vi "LOOP_pp3c_loadNext.vi"(0 "State Info In":T8={"Curr  tr"=0, "Curr (ms)"=0, "Cum (ms)"=0, "Run loop diff"=0, "Tone countdown (ms)"=0, "Countdown (ms)"=0, "Curr State"=enum."0 NULL", "Prev State"=enum."1 Habituation", "Rw"=FALSE, "Sw"=FALSE, "Tone\nGate"=FALSE, "Punish"=FALSE, "Current DAQ DO Int"=0, "Current Loaded Trial"={"Trial Type Number"=1, "Trial Type"=enum."GO", "Trial Weight"=100, "Shock (mA)"=0.3, "Duration (ms)"=0.25, "Sound Type"=enum."04 FM Sweep", "Stim P1"=4000.0, "Stim P2"=0.0, "Stim P3"=0.0, "Stim P4"=2000.0, "DAQ Amplitude (V)"=0.25}, "Total trials memo"=0, "State start cum memo (ms)"=0, "Last dur jump time memo (ms)"=0, "Last dur shock time memo (ms)"=0, "Tone repeat memo (ms)"=0, "Webcam on"=FALSE, "Webcam recording"=FALSE, "State update flag"=FALSE, "Last loaded shock voltage"=0.0, "Vid upd"=enum."0", "First time tone"=FALSE} {"Current DAQ DO Int" format="%016b"; "Current Loaded Trial"."DAQ Amplitude (V)" min=0.0 max=5.0 format="%_4g"; "Current Loaded Trial"."Shock (mA)" min=-1.0 max=5.0; "Current Loaded Trial"."Trial Weight" step=1; "Current Loaded Trial"."Duration (ms)" min=0.0 max=1.0; "Current Loaded Trial"."Trial Type Number" min=1 max=256 step=1}, 1 "Session param (dynamic)":T7={"Def M shock (uA)"=400.0, "Def F shock (uA)"=0.0}, 2 "Session List (Hidden variable)":u8[](array[numeric]), 3 "Trial Types":T1[](array[typedef])=[{"Trial Type Number"=1, "Trial Type"=enum."GO", "Trial Weight"=1, "Shock (mA)"=-1.0, "Duration (ms)"=250.0, "Sound Type"=enum."04 FM Sweep", "Stim P1"=4000.0, "Stim P2"=0.0, "Stim P3"=0.0, "Stim P4"=2000.0, "DAQ Amplitude (V)"=0.25}, {"Trial Type Number"=2, "Trial Type"=enum."NOGO", "Trial Weight"=1, "Shock (mA)"=-1.0, "Duration (ms)"=250.0, "Sound Type"=enum."04 FM Sweep", "Stim P1"=2000.0, "Stim P2"=0.0, "Stim P3"=0.0, "Stim P4"=4000.0, "DAQ Amplitude (V)"=0.25}] {"DAQ Amplitude (V)" min=0.0 max=5.0 format="%_4g"; "Shock (mA)" min=-1.0 max=5.0; "Trial Weight" step=1; "Duration (ms)" min=0.0 max=1.0; "Trial Type Number" min=1 max=256 step=1}, 5 "Daq config In":T4={"Sound AO"="Dev6/ao0", "Shock intesity AO"="Dev6/ao1", "Code_LED DO"="Dev6/port1:2", "Switch DI"="Dev6/port1/line0", "Webcam"="cam9", "Sound AO task"="", "Sound card task"=0, "Shock intensity AO task"="", "Code_LED DO task"="", "Switch DI task"="", "AO <=> Sound card"=FALSE, "Sound card"=0, "sample rate"=100000.0, "Variable shock"=TRUE, "Webcam on"=FALSE, "Waveform memo"={"t0"=timestamp(0 s since 1904-01-01), "dt"=1.0, "Y"=[]}, "Tone trigger"="PFI1", "Master-9 DO"="", "Master-9 DO task"="Dev6/port0/line5:7"} {"sample rate" min=8000.0; "Sound card task" format="%.0x"}, 7 "log queue in":refnum<queue>, 11 "error in (no error)":errorcluster) -> (4 "State Info Out":T8={"Curr  tr"=0, "Curr (ms)"=0, "Cum (ms)"=0, "Run loop diff"=0, "Tone countdown (ms)"=0, "Countdown (ms)"=0, "Curr State"=enum."0 NULL", "Prev State"=enum."1 Habituation", "Rw"=FALSE, "Sw"=FALSE, "Tone\nGate"=FALSE, "Punish"=FALSE, "Current DAQ DO Int"=0, "Current Loaded Trial"={"Trial Type Number"=1, "Trial Type"=enum."GO", "Trial Weight"=100, "Shock (mA)"=0.3, "Duration (ms)"=0.25, "Sound Type"=enum."04 FM Sweep", "Stim P1"=4000.0, "Stim P2"=0.0, "Stim P3"=0.0, "Stim P4"=2000.0, "DAQ Amplitude (V)"=0.25}, "Total trials memo"=0, "State start cum memo (ms)"=0, "Last dur jump time memo (ms)"=0, "Last dur shock time memo (ms)"=0, "Tone repeat memo (ms)"=0, "Webcam on"=FALSE, "Webcam recording"=FALSE, "State update flag"=FALSE, "Last loaded shock voltage"=0.0, "Vid upd"=enum."0", "First time tone"=FALSE} {"Current DAQ DO Int" format="%016b"; "Current Loaded Trial"."DAQ Amplitude (V)" min=0.0 max=5.0 format="%_4g"; "Current Loaded Trial"."Shock (mA)" min=-1.0 max=5.0; "Current Loaded Trial"."Trial Weight" step=1; "Current Loaded Trial"."Duration (ms)" min=0.0 max=1.0; "Current Loaded Trial"."Trial Type Number" min=1 max=256 step=1}, 8 "log queue out":refnum<queue>, 15 "error out":errorcluster)   [LabVIEW 2013]
doc: "This VI loads the next trial into \"current loaded trial\" in the State info, and applies approrpiate variable shock if applicable"
uses:
  CTL_pp3c_LoopState.ctl
  pp3_CTL_BehavioralState.ctl
  pp3_CTL_Trial.ctl
  pp3_CTL_TrialType.ctl
  labolabo2/waveforms/WFTypes.ctl
  pp3_CTL_SessionParamDynamic.ctl
  CTL_pp3c_DaqStatus.ctl
  <vilib>/userdefined/High Color/IMAQdx.ctl
  <vilib>/sound2/lvsound2.llb/Sound Output Task ID.ctl
  <vilib>/DAQmx/write.llb/DAQmx Write (Analog 1D DBL 1Chan NSamp).vi
  <vilib>/DAQmx/create/channels.llb/DAQmx Create Channel (AO-Voltage-Basic).vi
  <vilib>/DAQmx/configure/timing.llb/DAQmx Timing (Sample Clock).vi
  <vilib>/DAQmx/miscellaneous.llb/DAQmx Fill In Error Info.vi
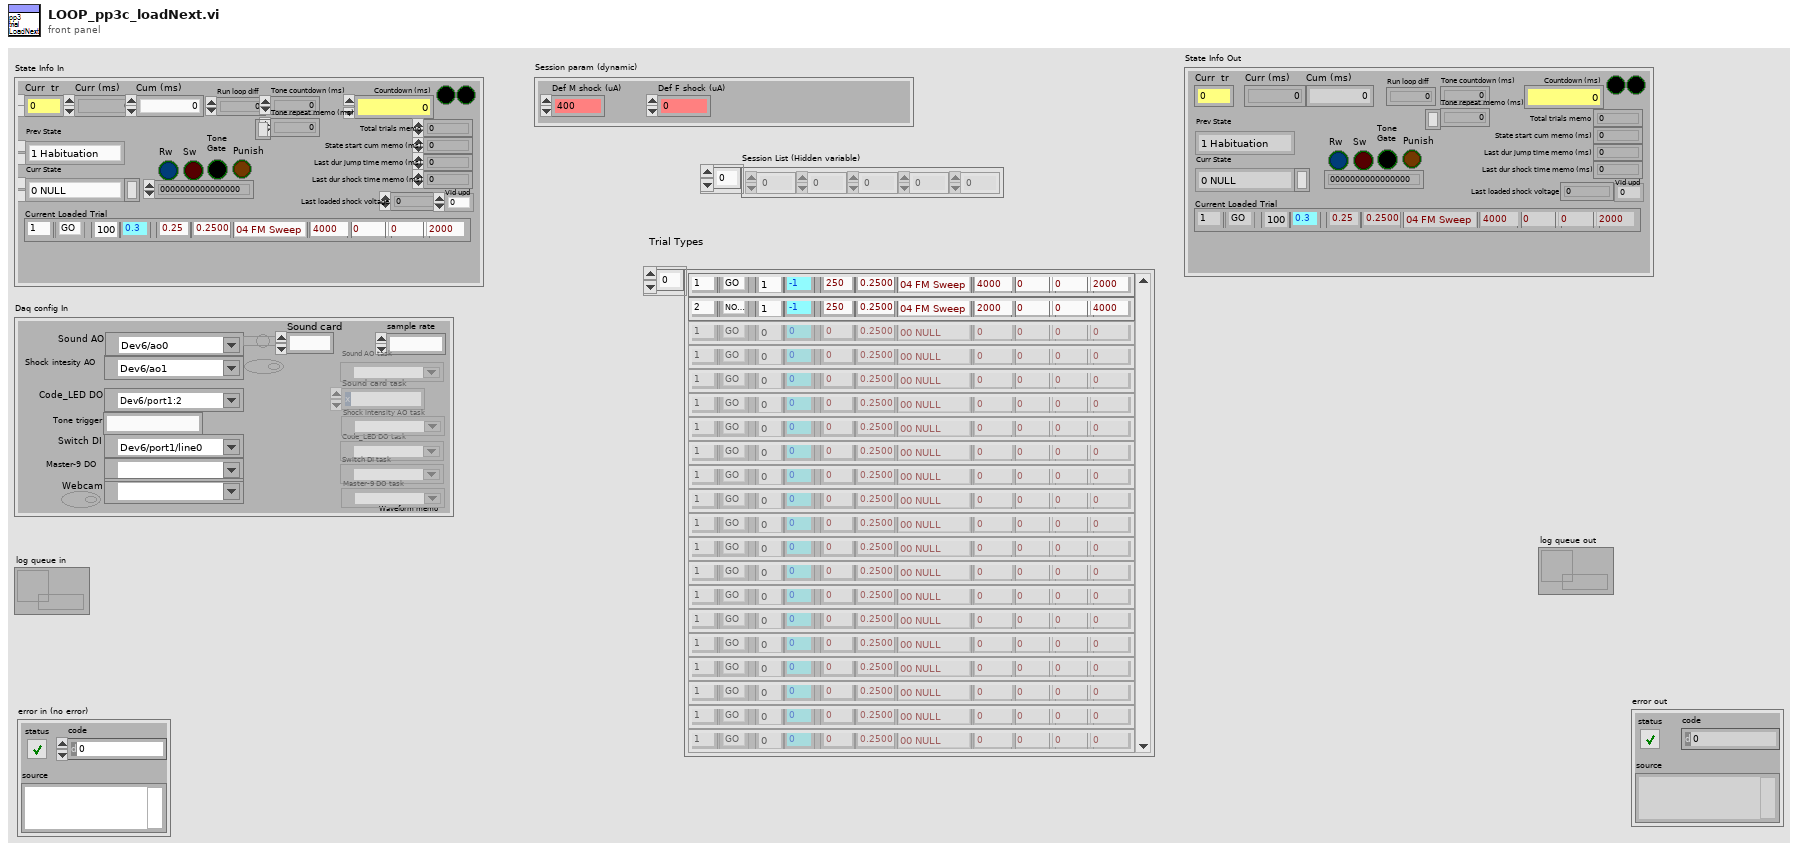
[diagram p1: front panel]
types:
  T1 = typedef "pp3_CTL_Trial.ctl" = cluster{"Trial Type Number":i16, "Trial Type":T2, "Trial Weight":u32, "Shock (mA)":dbl, "Duration (ms)":dbl, "Sound Type":T3, "Stim P1":dbl, "Stim P2":dbl, "Stim P3":dbl, "Stim P4":dbl, "DAQ Amplitude (V)":dbl}
  T2 = typedef "pp3_CTL_TrialType.ctl" = enum16{"OFF", "GO", "NOGO", "TEST"}
  T3 = typedef "WFTypes.ctl" = enum16{"00 NULL", "01 DC", "02 Noise", "03 Pure Tone", "04 FM Sweep"}
  T4 = typedef "CTL_pp3c_DaqStatus.ctl" = cluster{"Sound AO":tag, "Shock intesity AO":tag, "Code_LED DO":tag, "Switch DI":tag, "Webcam":T5, "Sound AO task":refnum<k21>, "Sound card task":T6, "Shock intensity AO task":refnum<k21>, "Code_LED DO task":refnum<k21>, "Switch DI task":refnum<k21>, "AO <=> Sound card":bool, "Sound card":u32, "sample rate":dbl, "Variable shock":bool, "Webcam on":bool, "Waveform memo":waveform(dbl), "Tone trigger":string, "Master-9 DO":tag, "Master-9 DO task":refnum<k21>}
  T5 = typedef "IMAQdx.ctl" = refnum<k21>
  T6 = typedef "Sound Output Task ID.ctl" = u32
  T7 = typedef "pp3_CTL_SessionParamDynamic.ctl" = cluster{"Def M shock (uA)":dbl, "Def F shock (uA)":dbl}
  T8 = typedef "CTL_pp3c_LoopState.ctl" = cluster{"Curr  tr":u16, "Curr (ms)":u32, "Cum (ms)":i64, "Run loop diff":i64, "Tone countdown (ms)":i64, "Countdown (ms)":i64, "Curr State":T9, "Prev State":T9, "Rw":bool, "Sw":bool, "Tone\nGate":bool, "Punish":bool, "Current DAQ DO Int":u16, "Current Loaded Trial":T1, "Total trials memo":i64, "State start cum memo (ms)":i64, "Last dur jump time memo (ms)":i64, "Last dur shock time memo (ms)":i64, "Tone repeat memo (ms)":i64, "Webcam on":bool, "Webcam recording":bool, "State update flag":bool, "Last loaded shock voltage":dbl, "Vid upd":enum16{"0", "1", "2", "3", "4", "5", "6", "7", "8", "9"}, "First time tone":bool}
  T9 = typedef "pp3_CTL_BehavioralState.ctl" = enum8{"0 NULL", "1 Habituation", "2 (Load Trial)", "3 Stay Period", "4 Load Audio/Click Delay", "5 GO Trial", "6 GO Jumped", "7 GO Timeout", "8 NOGO Trial", "9 NOGO Jumped", "10 NOGO Timeout", "11 TEST Trial", "12 TEST Jumped", "13 TEST Timeout", "14 Intertrial Interval", "15 Done"}
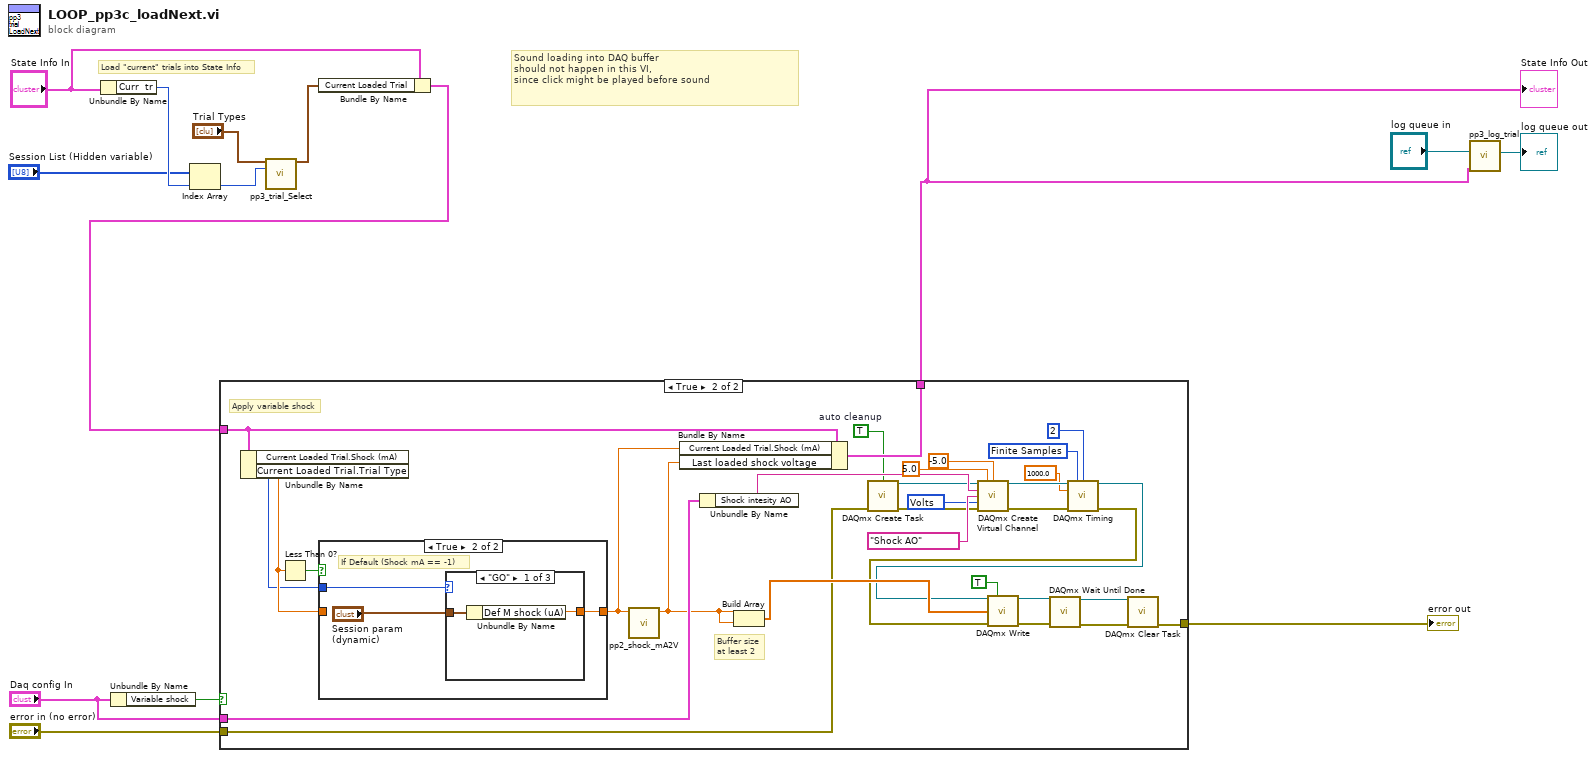
[diagram p0: block diagram]
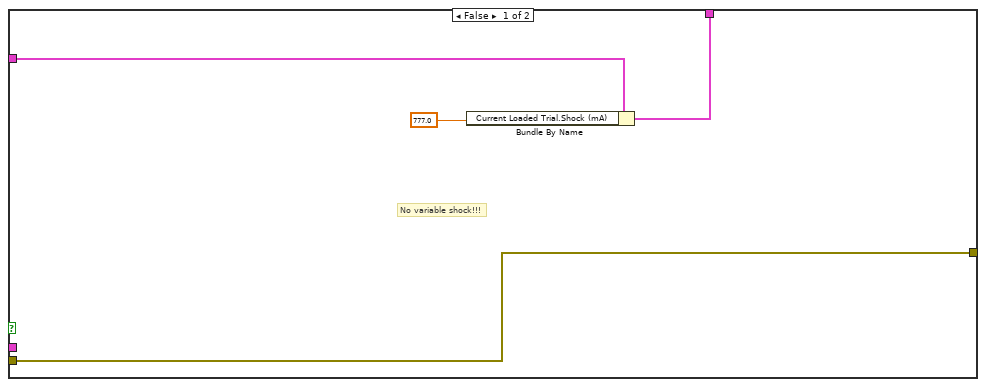
[diagram p2: hidden frame]
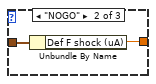
[diagram p4: hidden frame]
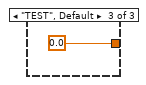
[diagram p5: hidden frame]
diagram:
  # "Load \"current\" trials into State Info"
  # "Sound loading into DAQ buffer\nshould not happen in this VI,\nsince click might be played before sound"
  n1 = Unbundle By Name("State Info In") -> ("Curr  tr"=w12:u16)
  n2 = Unbundle By Name("Daq config In") -> ("Variable shock"=w13:bool)
  n3 = Index Array(array="Session List (Hidden variable)", index=w12) -> (element=w9:u8)
  n4 = call "pp3_trial_Select.vi"("Trial Types"="Trial Types", "Code"=w9) -> ("Cluster 2"=w5:T1)  [unwired: 13 in]
  n5 = Bundle By Name(cluster="State Info In", "Current Loaded Trial"=w5) -> (w4:T8)
  n6 = case shown="True" w13 {
    tunnel: "Daq config In" -> [_ w35]
    tunnel: "error in (no error)" -> [w18 w24]
    tunnel: [w18 w32] -> w11
    tunnel: w4 -> [w16 w21]
    tunnel: [w17 w48] -> w1
    frame False {
      # "No variable shock!!!"
      n7 = Bundle By Name(cluster=w16, "Current Loaded Trial.Shock (mA)"=777.0) -> (w17:T8)
    }
    frame True {
      w25 = TRUE  # auto cleanup
      w38 = 10178 items=["Finite Samples"=10178, "Continuous Samples"=10123, "Hardware Timed Single Point"=12522] ("sample mode")
      w42 = 10348 items=["Volts"=10348, "From Custom Scale"=10065] ("units")
      # "Buffer size\nat least 2"
      # "Apply variable shock"
      n8 = Unbundle By Name(w21) -> ("Current Loaded Trial.Shock (mA)"=w20:dbl, "Current Loaded Trial.Trial Type"=w19:T2)
      n9 = Less Than 0?(x=w20) -> (x < 0?=w49:bool)
      n10 = case shown="True" w49 {
        tunnel: w19 -> [_ w53]
        tunnel: w20 -> [w50 _]
        tunnel: [w50 w51] -> w46
        frame False {
          # "If 0 or positive shock specification..."
        }
        frame True {
          # "If Default (Shock mA == -1)"
          n11 = case shown="\"GO\"" w53 {
            tunnel: "Session param (dynamic)" -> [w55 w57 _]
            tunnel: [w54 w56 0.0 ("Shock (mA)")] -> w51
            frame "GO" {
              n12 = Unbundle By Name(w55) -> ("Def M shock (uA)"=w54:dbl)
            }
            frame "NOGO" {
              n13 = Unbundle By Name(w57) -> ("Def F shock (uA)"=w56:dbl)
            }
            frame "TEST", Default {
            }
          }
        }
      }
      n14 = call "pp2_shock_mA2V.vi"("Shock (mA)"=w46) -> ("Shock (V)"=w29:dbl)  [unwired: 10 in]
      n15 = Bundle By Name(cluster=w21, "Current Loaded Trial.Shock (mA)"=w46, "Last loaded shock voltage"=w29) -> (w48:T8)
      n16 = Unbundle By Name(w35) -> ("Shock intesity AO"=w37:tag)
      n17 = Build Array(w29, w29) -> (w45:dbl[])
      n18 = call <vilib>:"DAQmx Create Task.vi"("auto cleanup"=w25, "error in"=w24) -> ("task out"=w23:refnum<k21>, "error out"=w22:errorcluster)  [unwired: 12 in]
      n19 = call-poly <vilib>:"DAQmx Create Virtual Channel.vi"("task in"=w23, "maximum value"=5.0, "minimum value"=-5.0, "physical channels"=w37, "name to assign"="Shock AO", "units"=w42, "error in"=w22) -> ("task out"=w40:refnum<k21>, "error out"=w39:errorcluster)  [unwired: 7 in]
      n20 = call-poly <vilib>:"DAQmx Timing.vi"("task/channels in"=w40, "sample mode"=w38, "samples per channel"=2, "rate"=1000.0, "error in"=w39) -> ("task out"=w31:refnum<k21>, "error out"=w30:errorcluster)  [unwired: 9 in]
      n21 = call-poly <vilib>:"DAQmx Write.vi"("task/channels in"=w31, "auto start"=TRUE, "data"=w45, "error in"=w30) -> ("task out"=w34:refnum<k21>, "error out"=w33:errorcluster)  [unwired: 9 in, 1 out]
      n22 = call <vilib>:"DAQmx Wait Until Done.vi"("task/channels in"=w34, "error in"=w33) -> ("task out"=w27:refnum<k21>, "error out"=w26:errorcluster)  [unwired: 12 in]
      n23 = call <vilib>:"DAQmx Clear Task.vi"("task in"=w27, "error in"=w26) -> ("error out"=w32:errorcluster)  [unwired: 13 in]
    }
  }
  "State Info Out" <- w1
  "error out" <- w11
  n24 = call "pp3_log_trial.vi"("State Info In"=w1, "queue in"="log queue in") -> ("queue out"=→"log queue out":refnum<queue>)  [unwired: 9 in]
